vi "constructor.vi"(8 "error in (no error)":errorcluster, 10 "Log Title":string) -> (0 "error out":errorcluster, 3 "Log out":refnum<class "Log.lvclass">)   [LabVIEW 2009, in "Tools.lvlib" / "xml.lvlib" / "Log.lvclass"]
uses:
  Log.lvclass
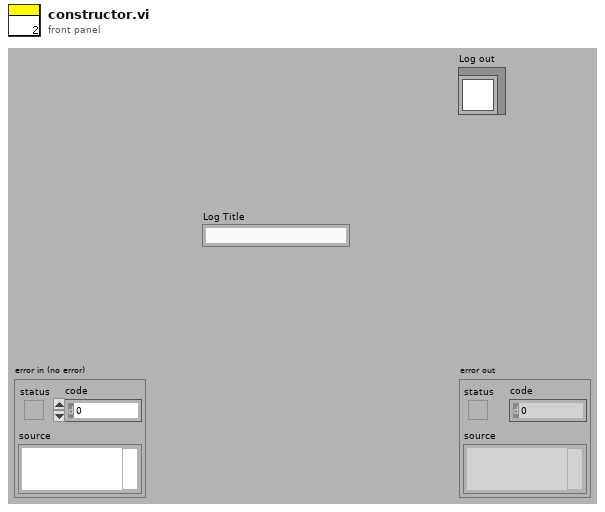
[diagram p1: front panel]
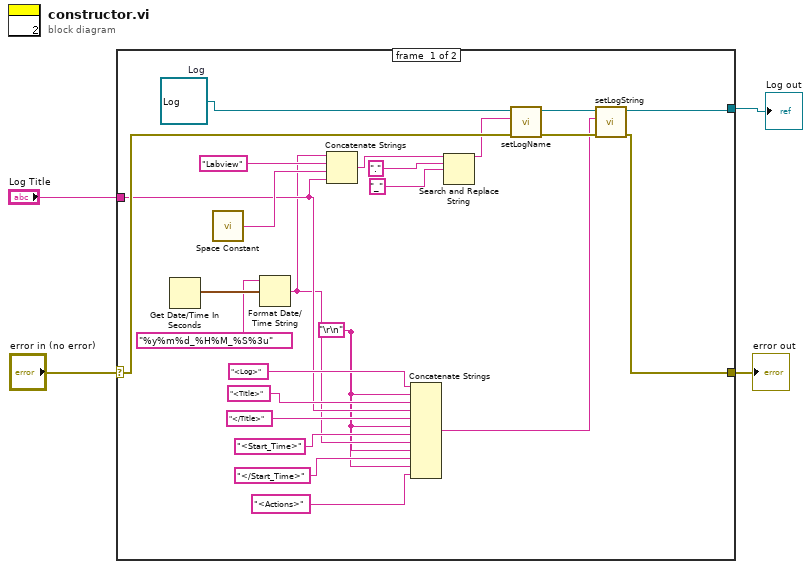
[diagram p0: block diagram]
diagram:
  n1 = case shown="No Error" "error in (no error)" {
    selector: "error in (no error)" -> [w24 w29]
    tunnel: [w27 w29] -> w3
    tunnel: [w26 _] -> w2
    tunnel: "Log Title" -> [w12 _]
    frame #0 {
      w25 = refnum<class "Log.lvclass"> refnum  # Log
      w7 = "\r\n"
      n2 = Get Date/Time In Seconds() -> (seconds since 1Jan1904=w28:timestamp)
      n3 = call <vilib>:"Space Constant.vi"() -> ("String"=w19:string)
      n4 = Format Date/Time String(time format string (%c)="%y%m%d_%H%M_%S%3u", seconds (now)=w28) -> (date/time string=w9:string)  [unwired: 1 in]
      n5 = Concatenate Strings(w9, "Labview", w19, w12) -> (w18:string)
      n6 = Concatenate Strings("<Log>", w7, "<Title>", w12, "</Title>", w7, "<Start_Time>", w9, w7, "</Start_Time>", w7, "<Actions>") -> (w5:string)
      n7 = Search and Replace String(input string=w18, search string=".", replace string="_") -> (result string=w15:string)  [unwired: 5 in, 3 out]
      n8 = call-dynamic "setLogName.vi"("error in (no error)"=w24, "logName"=w15, "Log.lvclass in"=w25) -> ("error out"=w22:errorcluster, "Log.lvclass out"=w23:refnum<class "Log.lvclass">)  [unwired: 7 in]
      n9 = call-dynamic "setLogString.vi"("error in (no error)"=w22, "logString"=w5, "Log.lvclass in"=w23) -> ("error out"=w27:errorcluster, "Log.lvclass out"=w26:refnum<class "Log.lvclass">)  [unwired: 7 in]
    }
    frame #1 {
    }
  }
  "error out" <- w3
  "Log out" <- w2
